vi "TSM_DataStream.vi"() -> ()   [LabVIEW 2020]
doc: "Output TSM raw Data Stream consiting of PGSI1, PGSI2, PGSIA, GPOH sentence via RS232 Port @ 38400 Baud. The stream data values are random numbers."
uses:
  <vilib>/Instr/_visa.llb/VISA Configure Serial Port (Instr).vi
  gVar_ECa2.vi
  gVar_ECa1.vi
  gVar_ECa4.vi
  gVar_ECa3.vi
panel:
  in  "R2 Only":bool
  in  "include GPOH":bool
  in  "Baud Rate":i32=38400
  in  "Factor of R1":dbl=2.0
  out "PGSIA":string="$PGSIA,+12.79,,,*77"
  out "PGSI2":string="$PGSI2,173850.000,0.00,+0.9,-0.00,+0.9*4A"
  in  "Temperature":string="23"
  in  "Pitch":string="2"
  in  "Roll":string="-3"
  in  "R4":dbl=12.0
  in  "R3":dbl=8.0
  out "PGSI1":string="$PGSI1,173850.000,0.00,+0.9,0.30,+0.9*3D\r\n"
  in  "R2":dbl=4.0
  in  "R1":dbl=1.0
  in  "Stopp":bool
  in  "COM Port":string="COM4"
  # "INPUT"
  # "OUTPUT"
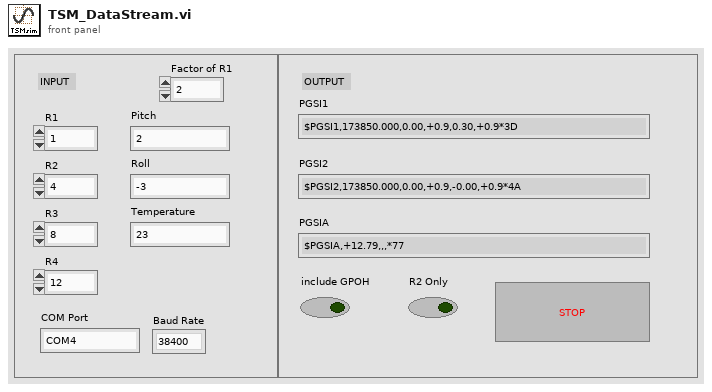
[diagram p1: front panel]
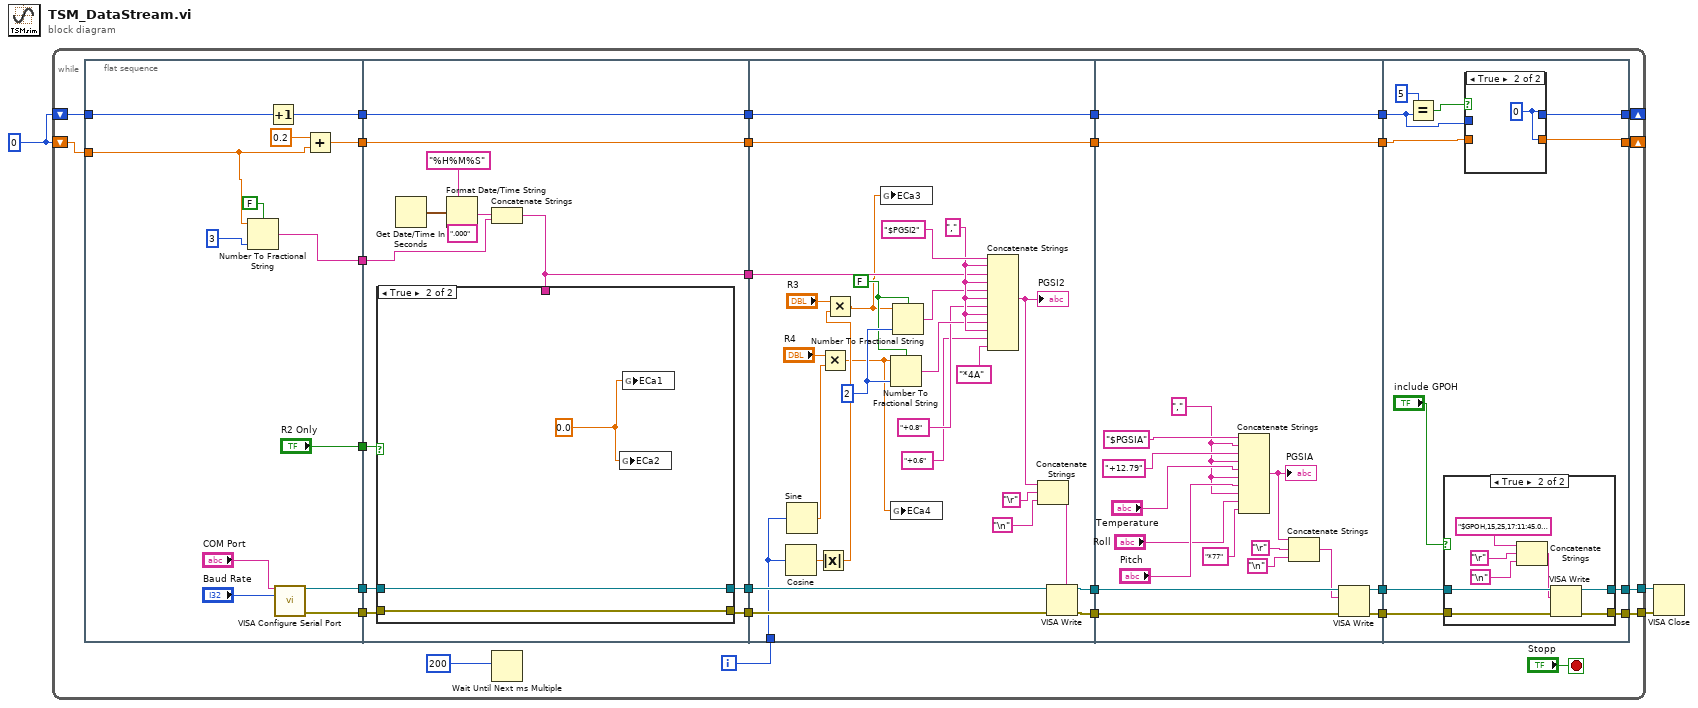
[diagram p0: block diagram]
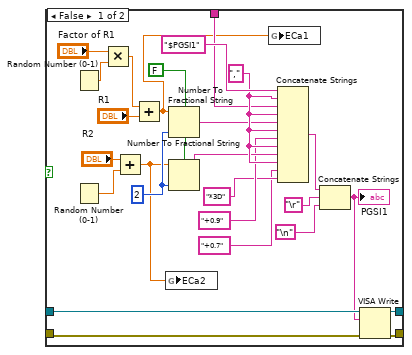
[diagram p2: hidden frame]
diagram:
  w1 = 0
  n1 = while {
    tunnel: [w25] -> w3
    tunnel: [w24] -> w2
    shift-right: [w12] -> _
    shift-left: w1 -> [w11]
    shift-right: [w5] -> _
    shift-left: w1 -> [w10]
    i -> [w18]
    stop <- "Stopp" stop-if-true
    n2 = flat-sequence {
      tunnel: [w43] -> w20
      tunnel: [w42] -> w19
      tunnel: ["R2 Only"] -> w17
      tunnel: [w38] -> w13
      tunnel: w11 -> [w35]
      tunnel: w10 -> [w37]
      tunnel: [w36] -> w6
      tunnel: [w34] -> w4
      tunnel: [w54] -> w31
      tunnel: [w53] -> w30
      tunnel: [w50] -> w21
      tunnel: w20 -> [w56]
      tunnel: w19 -> [w55]
      tunnel: w17 -> [w48]
      tunnel: [w47] -> w14
      tunnel: w13 -> [w47]
      tunnel: [w46] -> w7
      tunnel: w6 -> [w46]
      tunnel: w4 -> [w45]
      tunnel: w31 -> [w113]
      tunnel: w30 -> [w112]
      tunnel: [w111] -> w29
      tunnel: [w110] -> w28
      tunnel: w21 -> [w100]
      tunnel: w18 -> [w93]
      tunnel: [w87] -> w15
      tunnel: w14 -> [w87]
      tunnel: [w86] -> w8
      tunnel: w7 -> [w86]
      tunnel: w29 -> [w130]
      tunnel: w28 -> [w129]
      tunnel: [w128] -> w27
      tunnel: [w127] -> w26
      tunnel: [w115] -> w16
      tunnel: w15 -> [w115]
      tunnel: [w114] -> w9
      tunnel: w8 -> [w114]
      tunnel: w27 -> [w141]
      tunnel: w26 -> [w140]
      tunnel: [w139] -> w25
      tunnel: [w138] -> w24
      tunnel: [w131] -> w12
      tunnel: w16 -> [w132]
      tunnel: w9 -> [w134]
      tunnel: [w133] -> w5
      frame #0 {
        n3 = Number To Fractional String(use system decimal point (T)=FALSE, number=w35, precision (6)=3) -> (F-format string=w34:string)  [unwired: 1 in]
        n4 = Increment(x=w37) -> (x+1=w36:i32)
        n5 = call-poly "VISA Configure Serial Port"("VISA resource name"="COM Port", "baud rate (9600)"="Baud Rate") -> ("VISA resource name out"=w43:refnum<visa-resource-name>, "error out"=w42:errorcluster)  [unwired: 12 in]
        n6 = Add(x=0.2, y=w35) -> (x+y=w38:dbl)
      }
      frame #1 {
        (unwired) ".000"
        n7 = Get Date/Time In Seconds() -> (seconds since 1Jan1904=w51:timestamp)
        n8 = Format Date/Time String(time format string (%c)="%H%M%S", seconds (now)=w51) -> (date/time string=w49:string)  [unwired: 1 in]
        n9 = Concatenate Strings(w49, w45) -> (w50:string)
        n10 = case shown="True" w48 {
          tunnel: w56 -> [w82 w85]
          tunnel: w55 -> [w81 w84]
          tunnel: [w80 w85] -> w54
          tunnel: [w79 w84] -> w53
          tunnel: w50 -> [w60 _]
          frame False {
            w72 = ","
            w74 = 2
            w75 = FALSE
            n11 = Random Number (0-1)() -> (number: 0 to 1=w63:dbl)
            n12 = Random Number (0-1)() -> (number: 0 to 1=w77:dbl)
            n13 = Multiply(x="Factor of R1", y=w63) -> (x*y=w61:dbl)
            n14 = Add(x="R2", y=w77) -> (x+y=w57:dbl)
            n15 = Add(x=w61, y="R1") -> (x+y=w58:dbl)
            n16 = global write "gVar_ECa2.vi" "ECa2"(w57) -> ()
            n17 = Number To Fractional String(use system decimal point (T)=w75, number=w58, precision (6)=w74) -> (F-format string=w71:string)  [unwired: 1 in]
            n18 = Number To Fractional String(use system decimal point (T)=w75, number=w57, precision (6)=w74) -> (F-format string=w70:string)  [unwired: 1 in]
            n19 = global write "gVar_ECa1.vi" "ECa1"(w58) -> ()
            n20 = Concatenate Strings("$PGSI1", w72, w60, w72, w71, w72, "+0.9", w72, w70, w72, "+0.7", "*3D") -> (w67:string)
            n21 = Concatenate Strings(w67, "\r", "\n") -> (w66:string)
            "PGSI1" <- w66
            n22 = VISA Write(VISA resource name=w82, write buffer=w66, error in (no error)=w81) -> (VISA resource name out=w80:refnum<visa-resource-name>, error out=w79:errorcluster)  [unwired: 1 out]
          }
          frame True {
            w83 = 0.0
            n23 = global write "gVar_ECa2.vi" "ECa2"(w83) -> ()
            n24 = global write "gVar_ECa1.vi" "ECa1"(w83) -> ()
          }
        }
      }
      frame #2 {
        w102 = ","
        w104 = FALSE
        w106 = 2
        n25 = Cosine(x=w93) -> (cos(x)=w94:dbl)
        n26 = Sine(x=w93) -> (sin(x)=w92:dbl)
        n27 = Absolute Value(x=w94) -> (abs(x)=w91:dbl)
        n28 = Multiply(x="R4", y=w92) -> (x*y=w88:dbl)
        n29 = Multiply(x="R3", y=w91) -> (x*y=w89:dbl)
        n30 = global write "gVar_ECa3.vi" "ECa3"(w89) -> ()
        n31 = Number To Fractional String(use system decimal point (T)=w104, number=w88, precision (6)=w106) -> (F-format string=w98:string)  [unwired: 1 in]
        n32 = global write "gVar_ECa4.vi" "ECa4"(w88) -> ()
        n33 = Number To Fractional String(use system decimal point (T)=w104, number=w89, precision (6)=w106) -> (F-format string=w99:string)  [unwired: 1 in]
        n34 = Concatenate Strings("$PGSI2", w102, w100, w102, w99, w102, "+0.8", w102, w98, w102, "+0.6", "*4A") -> (w96:string)
        "PGSI2" <- w96
        n35 = Concatenate Strings(w96, "\r", "\n") -> (w108:string)
        n36 = VISA Write(VISA resource name=w113, write buffer=w108, error in (no error)=w112) -> (VISA resource name out=w111:refnum<visa-resource-name>, error out=w110:errorcluster)  [unwired: 1 out]
      }
      frame #3 {
        w119 = ","
        n37 = Concatenate Strings("$PGSIA", w119, "+12.79", w119, "Temperature", w119, "Pitch", w119, "Roll", "*77") -> (w116:string)
        "PGSIA" <- w116
        n38 = Concatenate Strings(w116, "\r", "\n") -> (w125:string)
        n39 = VISA Write(VISA resource name=w130, write buffer=w125, error in (no error)=w129) -> (VISA resource name out=w128:refnum<visa-resource-name>, error out=w127:errorcluster)  [unwired: 1 out]
      }
      frame #4 {
        n40 = Equal?(x=5, y=w134) -> (x = y?=w135:bool)
        n41 = case shown="True" "include GPOH" {
          tunnel: w141 -> [w146 w154]
          tunnel: w140 -> [w145 w153]
          tunnel: [w145 w152] -> w139
          tunnel: [w146 w151] -> w138
          frame False {
          }
          frame True {
            n42 = Concatenate Strings("$GPOH,15,25,17:11:45.000,A", "\r", "\n") -> (w148:string)
            n43 = VISA Write(VISA resource name=w154, write buffer=w148, error in (no error)=w153) -> (VISA resource name out=w151:refnum<visa-resource-name>, error out=w152:errorcluster)  [unwired: 1 out]
          }
        }
        n44 = case shown="True" w135 {
          tunnel: w134 -> [w143 _]
          tunnel: [w143 w144] -> w133
          tunnel: w132 -> [w142 _]
          tunnel: [w142 w144] -> w131
          frame False {
          }
          frame True {
            w144 = 0
          }
        }
      }
    }
    n45 = Wait Until Next ms Multiple(millisecond multiple=200) -> ()  [unwired: 1 out]
  }
  n46 = VISA Close(VISA resource name=w2, error in (no error)=w3) -> ()  [unwired: 1 out]
